vi "Copilot-Screen-(Controller).vi"() -> ()   [LabVIEW 2018]
uses:
  <vilib>/Instr/_visa.llb/VISA Configure Serial Port (Instr).vi
  <vilib>/Utility/inputDevices.llb/joystickAcquire.vi
  <vilib>/Utility/inputDevices.llb/closeJoystick.vi
  <vilib>/MakerHub/LINX/LMH-LINX.lvlib
panel:
  out "PH Reading":dbl format="%#_2f"
  in  "Horizontal Pulse 2":i32 caption="mp"
  out "Loop Rate (Hz)":u32
  in  "Temperature":bool
  in  "PH":bool
  in  "Metal":bool
  in  "R7":bool
  in  "R8":bool
  out "U Scaled":i32
  out "Teather Motor":bool
  out "Micro Backward":bool
  out "Micro Right":bool
  out "Micro Left":bool
  out "Micro Forward":bool
  out "CW":bool
  out "CCW":bool
  in  "MLED":bool
  in  "LMB":bool
  in  "LMF":bool
  in  "RMB":bool
  in  "RMF":bool
  in  "Reset":bool
  out "Seconds":i32
  out "Minutes":i32
  out "Timeout?":bool
  out "Horse Forward":bool
  out "Horse Backward":bool
  out "Down":bool
  out "Up":bool
  out "Backward":bool
  out "Left":bool
  out "Right":bool
  out "Forward":bool
  out "Horizontal Motion Case":string
  out "Horizontal %":i32
  out "Vertical Motion Case":string
  out "Vertical %":i32
  in  "Emergency Stop":bool
  out "X Scaled":i32
  out "Y Scaled":i32
  out "Z Scaled":i32
  out "ZR Scaled":i32
  out "axis info":T1
  out "button info":T2
  out "direction info":T3
  in  "R1":bool
  in  "ARM":bool
  in  "R3":bool
  in  "R4":bool
  in  "T1":bool
  in  "T2":bool
  in  "motion front left":bool
  in  "motion front right":bool
  in  "motion back right":bool
  in  "motion back left":bool
  in  "vertica front motors dir":bool
  in  "vertical back motors dir":bool
  in  "Horizontal Pulse 1":i32 caption="mp"
  in  "Vertical Pulse":i32 caption="vp"
  in  "To Arduino":string caption="Result"
  out "Sensor Reading":string
  out "error out":errorcluster
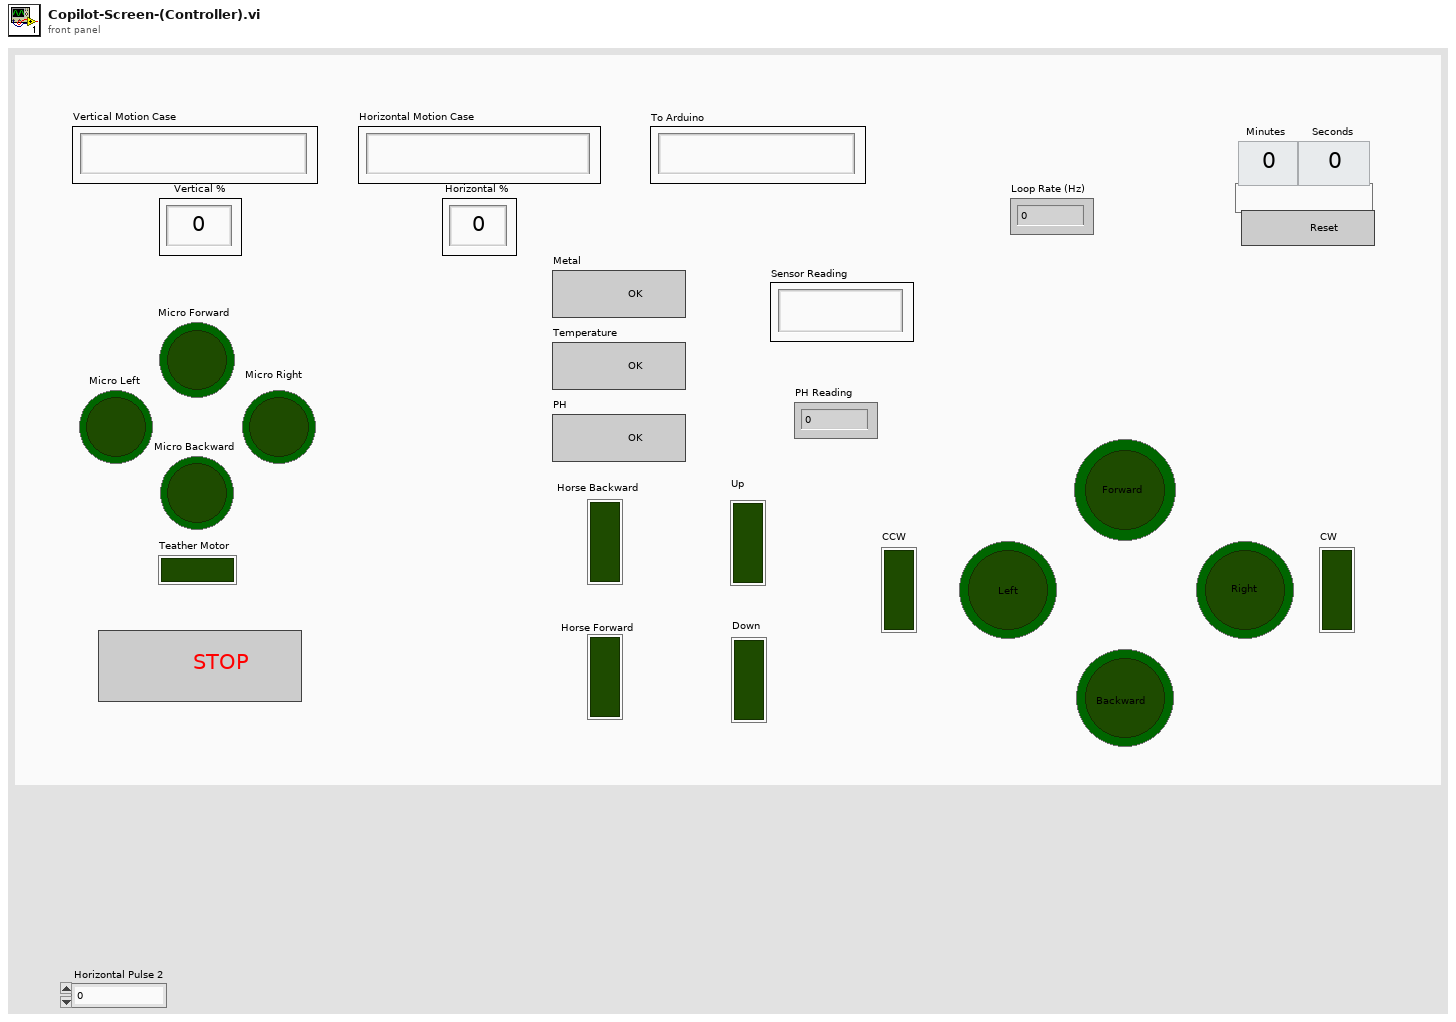
[diagram p1: front panel]
types:
  T1 = cluster{"X axis":i32, "Y axis":i32, "Z axis":i32, "X axis rotation":i32, "Y axis rotation":i32, "Z axis rotation":i32, "U axis":i32, "V axis":i32}
  T2 = cluster{"button 1":bool, "button 2":bool, "button 3":bool, "button 4":bool, "button 5":bool, "button 6":bool, "button 7":bool, "button 8":bool, "button 9":bool, "button 10":bool, "button 11":bool, "button 12":bool, "button 13":bool, "button 14":bool, "button 15":bool, "button 16":bool, "button 17":bool, "button 18":bool, "button 19":bool, "button 20":bool, "button 21":bool, "button 22":bool, "button 23":bool, "button 24":bool, "button 25":bool, "button 26":bool, "button 27":bool, "button 28":bool, "button 29":bool, "button 30":bool, "button 31":bool, "button 32":bool}
  T3 = cluster{"pov 1":i32, "pov 2":i32, "pov 3":i32, "pov 4":i32}
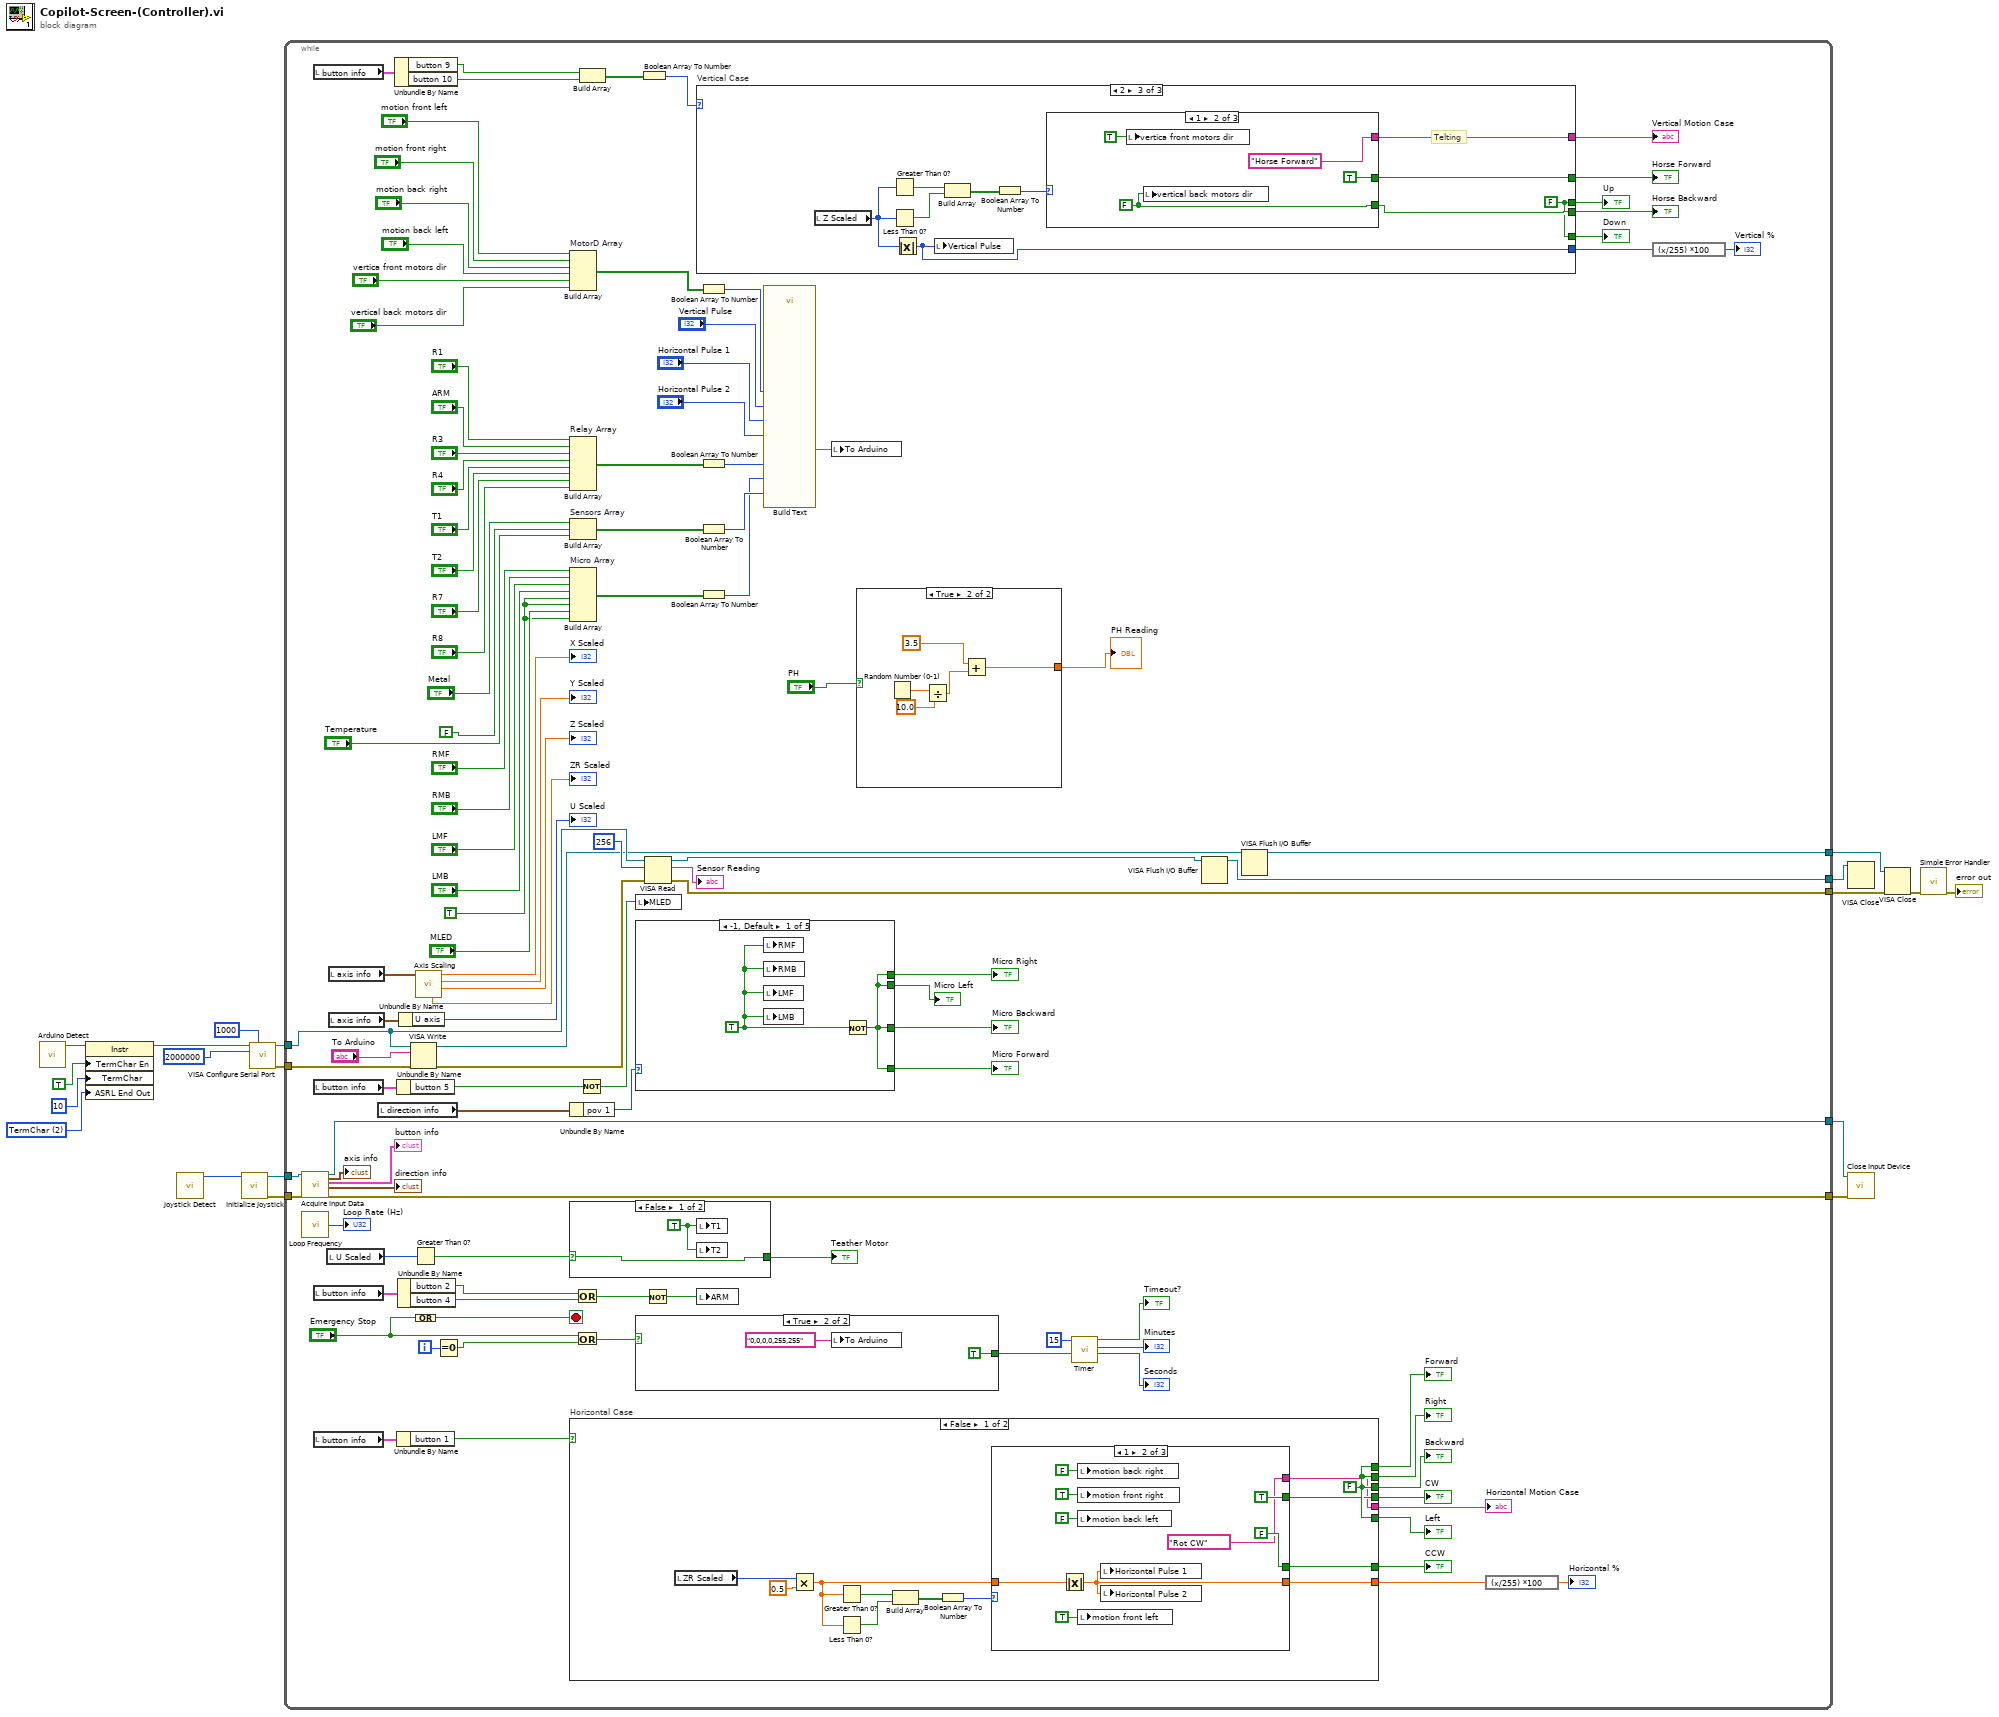
[diagram p0: block diagram]
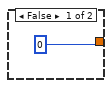
[diagram p2: hidden frame]
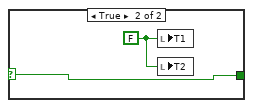
[diagram p3: hidden frame]
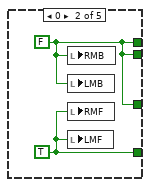
[diagram p4: hidden frame]
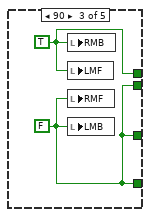
[diagram p5: hidden frame]
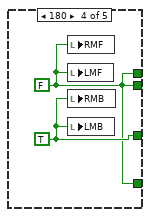
[diagram p6: hidden frame]
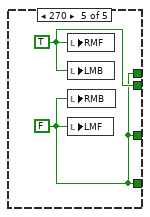
[diagram p7: hidden frame]
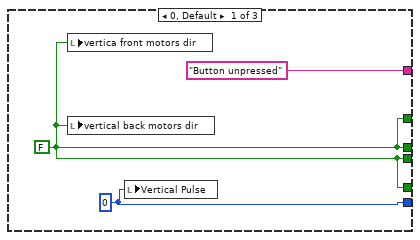
[diagram p8: hidden frame]
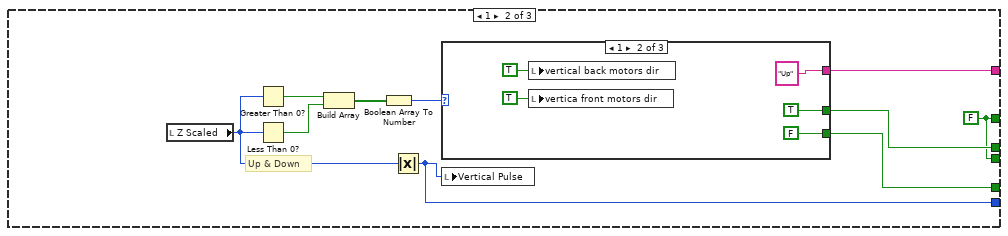
[diagram p9: hidden frame]
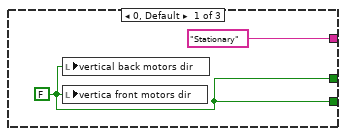
[diagram p10: hidden frame]
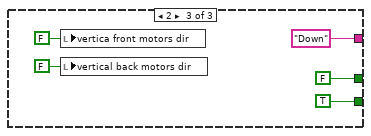
[diagram p11: hidden frame]
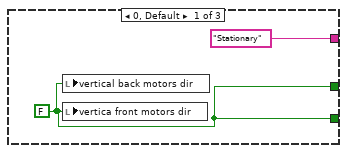
[diagram p12: hidden frame]
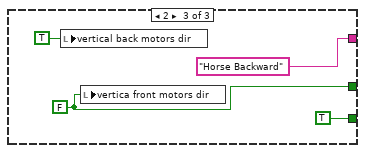
[diagram p13: hidden frame]
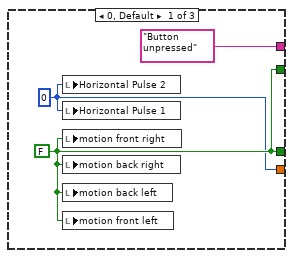
[diagram p14: hidden frame]
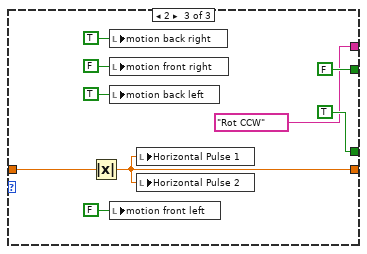
[diagram p15: hidden frame]
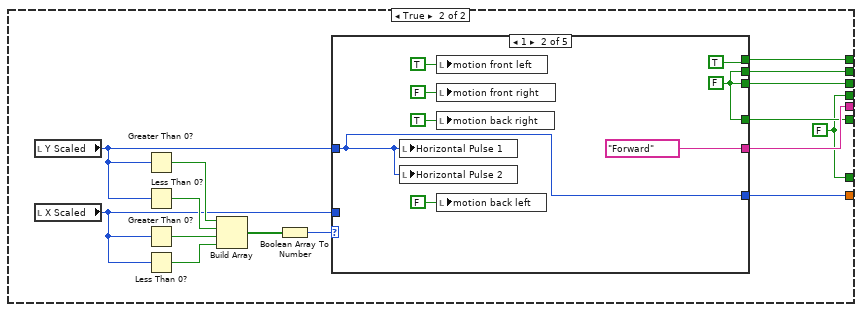
[diagram p16: hidden frame]
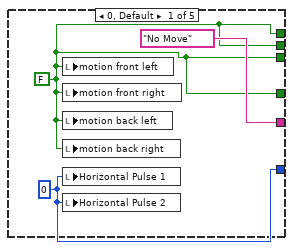
[diagram p17: hidden frame]
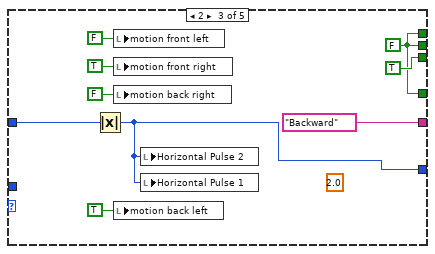
[diagram p18: hidden frame]
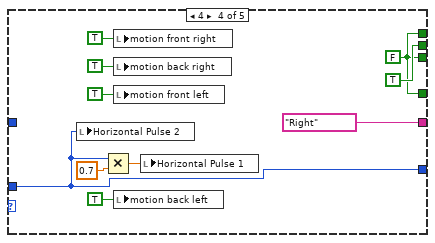
[diagram p19: hidden frame]
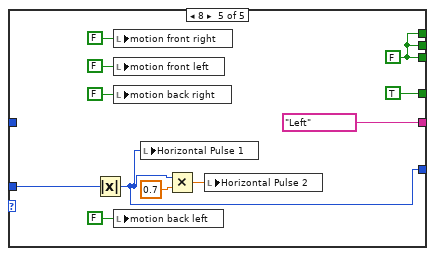
[diagram p20: hidden frame]
diagram:
  w5 = u16 2 items=["None", "Last Bit", "TermChar", "Break"] ("Serial Settings:End Mode for Writes")
  n1 = call "Arduino Detect.vi"() -> ("VISA Refnum out"=w2:refnum<visa-resource-name>)  [unwired: 9 in, 2 out]
  n2 = property class="Instr"(reference=w2, "TermChar En"=TRUE ("Message Based Settings:Termination Character Enable"), "TermChar"=u8 10 ("Message Based Settings:Termination Character"), "ASRL End Out"=w5) -> (reference out=w3:refnum<visa-resource-name>)  [unwired: 1 in, 1 out]
  n3 = call "Joystick Detect.vi"() -> ("ID"=w1:i32)  [unwired: 11 in]
  n4 = call <vilib>:"Initialize Joystick.vi"("device index"=w1) -> ("error out"=w10:errorcluster, "device ID"=w11:refnum<k1>)  [unwired: 9 in]
  n5 = call-poly "VISA Configure Serial Port"("VISA resource name"=w3, "timeout (10sec)"=u32 1000, "baud rate (9600)"=u32 2000000 ("baud rate")) -> ("VISA resource name out"=w15:refnum<visa-resource-name>, "error out"=w14:errorcluster)  [unwired: 11 in]
  n6 = while {
    tunnel: w15 -> [w88]
    tunnel: w14 -> [w130]
    tunnel: [w87] -> w13
    tunnel: [w129] -> w12
    tunnel: w11 -> [w111]
    tunnel: w10 -> [w110]
    tunnel: [w109] -> w9
    tunnel: [w108] -> w8
    tunnel: [w79] -> w7
    i -> [w85]
    stop <- w104 stop-if-true
    w23 = TRUE
    n7 = call-poly <vilib>:"Acquire Input Data.vi"("device ID"=w111, "error in (no error)"=w110) -> ("device ID"=w108:refnum<k1>, "axis info"=→"axis info":T1, "button info"=→"button info":T2, "direction info"=→"direction info":T3, "error out"=w109:errorcluster)  [unwired: 13 in]
    n8 = call <vilib>:"Loop Frequency.vi"() -> ("Loop Rate (Hz)"=→"Loop Rate (Hz)":u32)
    n9 = local read "button info"() -> (w100:T2)
    n10 = local read "button info"() -> (w44:T2)
    n11 = local read "button info"() -> (w89:T2)
    n12 = local read "button info"() -> (w93:T2)
    n13 = local read "U Scaled"() -> (w49:i32)
    n14 = local read "axis info"() -> (w74:T1)
    n15 = local read "axis info"() -> (w40:T1)
    n16 = local read "direction info"() -> (w59:T3)
    n17 = Unbundle By Name(w100) -> ("button 9"=w99:bool, "button 10"=w98:bool)
    n18 = Unbundle By Name(w44) -> ("button 5"=w43:bool)
    n19 = Unbundle By Name(w93) -> ("button 1"=w53:bool)
    n20 = Unbundle By Name(w89) -> ("button 2"=w82:bool, "button 4"=w81:bool)
    n21 = Unbundle By Name(w40) -> ("U axis"=→"U Scaled":i32)
    n22 = VISA Write(VISA resource name=w88, write buffer="To Arduino", error in (no error)=w130) -> (VISA resource name out=w86:refnum<visa-resource-name>, error out=w132:errorcluster)  [unwired: 1 out]
    n23 = Greater Than 0?(x=w49) -> (x > 0?=w46:bool)
    n24 = call "Axis Scaling.vi"("axis info"=w74) -> ("Scalar 2"=→"Z Scaled":dbl, "Scalar"=→"Y Scaled":dbl, "Scalar 4"=→"X Scaled":dbl, "Scalar 3"=→"ZR Scaled":dbl)  [unwired: 6 in, 1 out]
    n25 = Compound Arithmetic op=OR("Emergency Stop") -> (w104:bool)
    n26 = Equal To 0?(x=w85) -> (x = 0?=w105:bool)
    n27 = Build Array "MotorD Array"("motion front left", "motion front right", "motion back right", "motion back left", "vertica front motors dir", "vertical back motors dir") -> (w126:bool[])
    n28 = Build Array "Relay Array"("R1", "ARM", "R3", "R4", "T1", "T2", "R7", "R8") -> (w118:bool[])
    n29 = Build Array "Sensors Array"("Metal", FALSE ("element"), "Temperature") -> (w38:bool[])
    n30 = Build Array "Micro Array"("RMF", "RMB", "LMF", "LMB", w23, w23, "MLED", w23) -> (w29:bool[])
    n31 = Unbundle By Name(w59) -> ("pov 1"=w58:i32)
    n32 = case shown="False" w46 {
      selector: w46 -> [w140 w142]
      tunnel: [w140 w142] -> w45
      frame False {
        w139 = TRUE ("LMF")
        n33 = local write "T1"(w139) -> ()
        n34 = local write "T2"(w139) -> ()
      }
      frame True {
        w141 = FALSE ("LMF")
        n35 = local write "T1"(w141) -> ()
        n36 = local write "T2"(w141) -> ()
      }
    }
    "Teather Motor" <- w45
    n37 = case "Horizontal Case" shown="False" w53 {
      tunnel: [w201 w245] -> w96
      tunnel: [w202 w236] -> w95
      tunnel: [w209 w234] -> w64
      tunnel: [w209 w233] -> w63
      tunnel: [w209 w232] -> w62
      tunnel: [w209 w235] -> w61
      tunnel: [w204 w231] -> w52
      tunnel: [w203 w231] -> w51
      frame False {
        w209 = FALSE ("motion back left")
        n38 = local read "ZR Scaled"() -> (w200:i32)
        n39 = Multiply(x=w200, y=0.5) -> (x*y=w199:dbl)
        n40 = Greater Than 0?(x=w199) -> (x > 0?=w207:bool)
        n41 = Less Than 0?(x=w199) -> (x < 0?=w208:bool)
        n42 = Build Array(w207, w208) -> (w205:bool[])
        n43 = Boolean Array To Number(Boolean array=w205) -> (number=w206:u32)
        n44 = case shown="1" w206 {
          tunnel: [w210 w213 w222] -> w202
          tunnel: [w212 FALSE TRUE] -> w204
          tunnel: [w212 TRUE FALSE] -> w203
          tunnel: w199 -> [_ w215 w224]
          tunnel: ["Button unpressed" ("String 2") "Rot CW" ("String 2") "Rot CCW" ("String 2")] -> w201
          frame 0, Default {
            w212 = FALSE
            w210 = 0 ("Motion Pulse")
            n45 = local write "Horizontal Pulse 2"(w210) -> ()
            n46 = local write "Horizontal Pulse 1"(w210) -> ()
            n47 = local write "motion front right"(w212) -> ()
            n48 = local write "motion back right"(w212) -> ()
            n49 = local write "motion back left"(w212) -> ()
            n50 = local write "motion front left"(w212) -> ()
          }
          frame 1 {
            n51 = Absolute Value(x=w215) -> (abs(x)=w213:dbl)
            n52 = local write "motion back right"(FALSE) -> ()
            n53 = local write "motion front right"(TRUE) -> ()
            n54 = local write "motion back left"(FALSE) -> ()
            n55 = local write "motion front left"(TRUE) -> ()
            n56 = local write "Horizontal Pulse 1"(w213) -> ()
            n57 = local write "Horizontal Pulse 2"(w213) -> ()
          }
          frame 2 {
            n58 = Absolute Value(x=w224) -> (abs(x)=w222:dbl)
            n59 = local write "motion back right"(TRUE) -> ()
            n60 = local write "motion front right"(FALSE) -> ()
            n61 = local write "motion back left"(TRUE) -> ()
            n62 = local write "motion front left"(FALSE) -> ()
            n63 = local write "Horizontal Pulse 1"(w222) -> ()
            n64 = local write "Horizontal Pulse 2"(w222) -> ()
          }
        }
      }
      frame True {
        w231 = FALSE ("motion back left")
        n65 = local read "Y Scaled"() -> (w238:i32)
        n66 = local read "X Scaled"() -> (w237:i32)
        n67 = Greater Than 0?(x=w238) -> (x > 0?=w243:bool)
        n68 = Less Than 0?(x=w238) -> (x < 0?=w242:bool)
        n69 = Greater Than 0?(x=w237) -> (x > 0?=w241:bool)
        n70 = Less Than 0?(x=w237) -> (x < 0?=w240:bool)
        n71 = Build Array(w243, w242, w241, w240) -> (w239:bool[])
        n72 = Boolean Array To Number(Boolean array=w239) -> (number=w244:u32)
        n73 = case shown="1" w244 {
          tunnel: ["No Move" ("String 2") "Forward" ("String 2") "Backward" ("String 2") "Right" ("String 2") "Left" ("String 2")] -> w245
          tunnel: w238 -> [_ w249 w264 _ _]
          tunnel: w237 -> [_ _ _ w267 w285]
          tunnel: [w246 w249 w257 w267 w276] -> w236
          tunnel: [w247 w250 w258 w269 TRUE] -> w235
          tunnel: [w247 w250 TRUE w269 w279] -> w234
          tunnel: [w247 TRUE w258 w269 w279] -> w233
          tunnel: [w247 w250 w258 TRUE w279] -> w232
          frame 0, Default {
            w247 = FALSE
            w246 = 0 ("Motion Pulse")
            n74 = local write "motion front left"(w247) -> ()
            n75 = local write "motion front right"(w247) -> ()
            n76 = local write "motion back left"(w247) -> ()
            n77 = local write "motion back right"(w247) -> ()
            n78 = local write "Horizontal Pulse 1"(w246) -> ()
            n79 = local write "Horizontal Pulse 2"(w246) -> ()
          }
          frame 1 {
            w250 = FALSE
            n80 = local write "Horizontal Pulse 1"(w249) -> ()
            n81 = local write "Horizontal Pulse 2"(w249) -> ()
            n82 = local write "motion front left"(TRUE) -> ()
            n83 = local write "motion front right"(FALSE) -> ()
            n84 = local write "motion back right"(TRUE) -> ()
            n85 = local write "motion back left"(FALSE) -> ()
          }
          frame 2 {
            (unwired) 2.0 ("y")
            w258 = FALSE
            n86 = Absolute Value(x=w264) -> (abs(x)=w257:i32)
            n87 = local write "motion front left"(FALSE) -> ()
            n88 = local write "motion front right"(TRUE) -> ()
            n89 = local write "motion back right"(FALSE) -> ()
            n90 = local write "motion back left"(TRUE) -> ()
            n91 = local write "Horizontal Pulse 2"(w257) -> ()
            n92 = local write "Horizontal Pulse 1"(w257) -> ()
          }
          frame 4 {
            w269 = FALSE
            n93 = local write "Horizontal Pulse 2"(w267) -> ()
            n94 = Multiply(x=w267, y=0.7) -> (x*y=w266:dbl)
            n95 = local write "motion front right"(TRUE) -> ()
            n96 = local write "motion back right"(TRUE) -> ()
            n97 = local write "motion front left"(TRUE) -> ()
            n98 = local write "motion back left"(TRUE) -> ()
            n99 = local write "Horizontal Pulse 1"(w266) -> ()
          }
          frame 8 {
            w279 = FALSE
            n100 = Absolute Value(x=w285) -> (abs(x)=w276:i32)
            n101 = local write "motion front right"(FALSE) -> ()
            n102 = local write "motion front left"(FALSE) -> ()
            n103 = local write "motion back right"(FALSE) -> ()
            n104 = local write "motion back left"(FALSE) -> ()
            n105 = local write "Horizontal Pulse 1"(w276) -> ()
            n106 = Multiply(x=w276, y=0.7) -> (x*y=w277:dbl)
            n107 = local write "Horizontal Pulse 2"(w277) -> ()
          }
        }
      }
    }
    "Horizontal Motion Case" <- w96
    "Forward" <- w63
    "Right" <- w62
    "Left" <- w61
    "Backward" <- w64
    "CCW" <- w52
    "CW" <- w51
    n108 = Or(x=w82, y=w81) -> (x .or. y?=w60:bool)
    n109 = Or(x="Emergency Stop", y=w105) -> (x .or. y?=w107:bool)
    n110 = Not(x=w43) -> (.not. x?=w42:bool)
    n111 = Build Array(w99, w98) -> (w97:bool[])
    n112 = local write "MLED"(w42) -> ()
    n113 = case shown="-1, Default" w58 {
      tunnel: [w143 w146 w147 w149 w151] -> w57
      tunnel: [w143 w145 w148 w149 w151] -> w56
      tunnel: [w143 w145 w147 w150 w151] -> w55
      tunnel: [w143 w145 w147 w149 w152] -> w54
      frame -1, Default {
        w144 = TRUE ("RMF")
        n114 = local write "RMF"(w144) -> ()
        n115 = local write "RMB"(w144) -> ()
        n116 = local write "LMF"(w144) -> ()
        n117 = local write "LMB"(w144) -> ()
        n118 = Not(x=w144) -> (.not. x?=w143:bool)
      }
      frame 0 {
        w145 = FALSE ("RMF")
        w146 = TRUE ("RMF")
        n119 = local write "RMB"(w145) -> ()
        n120 = local write "LMB"(w145) -> ()
        n121 = local write "RMF"(w146) -> ()
        n122 = local write "LMF"(w146) -> ()
      }
      frame 90 {
        w147 = FALSE ("RMF")
        w148 = TRUE ("LMF")
        n123 = local write "RMB"(w148) -> ()
        n124 = local write "LMF"(w148) -> ()
        n125 = local write "RMF"(w147) -> ()
        n126 = local write "LMB"(w147) -> ()
      }
      frame 180 {
        w149 = FALSE ("LMF")
        w150 = TRUE ("RMB")
        n127 = local write "RMF"(w149) -> ()
        n128 = local write "LMF"(w149) -> ()
        n129 = local write "RMB"(w150) -> ()
        n130 = local write "LMB"(w150) -> ()
      }
      frame 270 {
        w151 = FALSE ("RMB")
        w152 = TRUE ("RMF")
        n131 = local write "RMF"(w152) -> ()
        n132 = local write "LMB"(w152) -> ()
        n133 = local write "RMB"(w151) -> ()
        n134 = local write "LMF"(w151) -> ()
      }
    }
    "Micro Forward" <- w57
    "Micro Left" <- w54
    "Micro Right" <- w56
    "Micro Backward" <- w55
    n135 = case shown="True" w107 {
      tunnel: ["Reset" TRUE ("Reset")] -> w69
      frame False {
      }
      frame True {
        n136 = local write "To Arduino"("0,0,0,0,255,255" ("write string")) -> ()
      }
    }
    n137 = Boolean Array To Number(Boolean array=w97) -> (number=w83:u32)
    n138 = VISA Read(VISA resource name=w88, byte count=u32 256, error in (no error)=w132) -> (VISA resource name out=w80:refnum<visa-resource-name>, read buffer=→"Sensor Reading":string, error out=w129:errorcluster)  [unwired: 1 out]
    n139 = Not(x=w60) -> (.not. x?=w50:bool)
    n140 = case "Vertical Case" shown="2" w83 {
      tunnel: ["Button unpressed" ("String 3") w164 w182] -> w103
      tunnel: [w154 w163 w181] -> w102
      tunnel: [w153 w158 w178] -> w78
      tunnel: [w153 w157 w178] -> w77
      tunnel: [w153 w156 w180] -> w76
      tunnel: [w153 w156 w179] -> w75
      frame 0, Default {
        w153 = FALSE ("vertica front motors dir")
        w154 = 0 ("Vertical Pulse")
        n141 = local write "vertica front motors dir"(w153) -> ()
        n142 = local write "vertical back motors dir"(w153) -> ()
        n143 = local write "Vertical Pulse"(w154) -> ()
      }
      frame 1 {
        w156 = FALSE ("Up")
        # "Up & Down"
        n144 = local read "Z Scaled"() -> (w159:i32)
        n145 = Greater Than 0?(x=w159) -> (x > 0?=w160:bool)
        n146 = Less Than 0?(x=w159) -> (x < 0?=w161:bool)
        n147 = Build Array(w160, w161) -> (w162:bool[])
        n148 = Boolean Array To Number(Boolean array=w162) -> (number=w165:u32)
        n149 = Absolute Value(x=w159) -> (abs(x)=w163:i32)
        n150 = case shown="1" w165 {
          tunnel: ["Stationary" ("f") "Up" ("String 3") "Down" ("String 3")] -> w164
          tunnel: [w166 TRUE ("Up") FALSE ("Down")] -> w158
          tunnel: [w166 FALSE ("Up") TRUE ("Down")] -> w157
          frame 0, Default {
            w166 = FALSE ("vertica front motors dir")
            n151 = local write "vertical back motors dir"(w166) -> ()
            n152 = local write "vertica front motors dir"(w166) -> ()
          }
          frame 1 {
            n153 = local write "vertical back motors dir"(TRUE ("vertica front motors dir")) -> ()
            n154 = local write "vertica front motors dir"(TRUE ("vertica front motors dir")) -> ()
          }
          frame 2 {
            n155 = local write "vertica front motors dir"(FALSE ("vertica front motors dir")) -> ()
            n156 = local write "vertical back motors dir"(FALSE ("vertical back motors dir")) -> ()
          }
        }
        n157 = local write "Vertical Pulse"(w163) -> ()
      }
      frame 2 {
        w178 = FALSE ("vertica front motors dir")
        # "Telting"
        n158 = local read "Z Scaled"() -> (w187:i32)
        n159 = Greater Than 0?(x=w187) -> (x > 0?=w185:bool)
        n160 = Less Than 0?(x=w187) -> (x < 0?=w184:bool)
        n161 = Absolute Value(x=w187) -> (abs(x)=w181:i32)
        n162 = local write "Vertical Pulse"(w181) -> ()
        n163 = Build Array(w185, w184) -> (w183:bool[])
        n164 = Boolean Array To Number(Boolean array=w183) -> (number=w186:u32)
        n165 = case shown="1" w186 {
          tunnel: ["Stationary" ("f") "Horse Forward" ("String 3") "Horse Backward" ("String 3")] -> w182
          tunnel: [w188 TRUE ("Horse Forward") w194] -> w180
          tunnel: [w188 w190 TRUE ("Horse Backward")] -> w179
          frame 0, Default {
            w188 = FALSE ("vertica front motors dir")
            n166 = local write "vertical back motors dir"(w188) -> ()
            n167 = local write "vertica front motors dir"(w188) -> ()
          }
          frame 1 {
            w190 = FALSE ("vertica front motors dir")
            n168 = local write "vertica front motors dir"(TRUE ("vertica front motors dir")) -> ()
            n169 = local write "vertical back motors dir"(w190) -> ()
          }
          frame 2 {
            w194 = FALSE ("vertica front motors dir")
            n170 = local write "vertical back motors dir"(TRUE ("vertica front motors dir")) -> ()
            n171 = local write "vertica front motors dir"(w194) -> ()
          }
        }
      }
    }
    "Vertical Motion Case" <- w103
    "Up" <- w78
    "Down" <- w77
    "Horse Forward" <- w76
    "Horse Backward" <- w75
    n172 = local write "ARM"(w50) -> ()
    n173 = Boolean Array To Number(Boolean array=w126) -> (number=w31:u32)
    n174 = Boolean Array To Number(Boolean array=w118) -> (number=w32:u32)
    n175 = Boolean Array To Number(Boolean array=w38) -> (number=w34:u32)
    n176 = Boolean Array To Number(Boolean array=w29) -> (number=w33:u32)
    n177 = call "Build Text"("MotorD"=w31, "Micro"=w33, "VP"="Vertical Pulse", "HP1"="Horizontal Pulse 1", "HP2"="Horizontal Pulse 2", "Relay"=w32, "Sensors"=w34) -> ("Result"=w92:string)  [unwired: 7 in, 1 out]
    n178 = local write "To Arduino"(w92) -> ()
    n179 = case shown="True" "PH" {
      tunnel: [0 w134] -> w20
      frame False {
      }
      frame True {
        n180 = Random Number (0-1)() -> (number: 0 to 1=w136:dbl)
        n181 = Divide(x=w136, y=10.0) -> (x/y=w137:dbl)
        n182 = Add(x=3.5, y=w137) -> (x+y=w134:dbl)
      }
    }
    "PH Reading" <- w20
    n183 = call "Timer.vi"("My Minutes"=15, "Reset"=w69) -> ("Timeout?"=→"Timeout?":bool, "Minutes"=→"Minutes":i32, "Seconds"=→"Seconds":i32)  [unwired: 6 in]
    n184 = VISA Flush I/O Buffer(VISA resource name=w80) -> (VISA resource name out=w79:refnum<visa-resource-name>)  [unwired: 2 in, 1 out]
    n185 = VISA Flush I/O Buffer(VISA resource name=w86) -> (VISA resource name out=w87:refnum<visa-resource-name>)  [unwired: 2 in, 1 out]
    n186 = expression code="(x/255) *100"(w95) -> (→"Horizontal %":dbl)
    n187 = expression code="(x/255) *100"(w102) -> (→"Vertical %":i32)
  }
  n188 = VISA Close(VISA resource name=w7) -> ()  [unwired: 1 in, 1 out]
  n189 = call-poly <vilib>:"Close Input Device.vi"("error in (no error)"=w9, "device ID"=w8) -> ()  [unwired: 8 in, 1 out]
  n190 = VISA Close(VISA resource name=w13, error in (no error)=w12) -> (error out=w18:errorcluster)
  n191 = call <vilib>:"Simple Error Handler.vi"("error in (no error)"=w18) -> ("error out"=→"error out":errorcluster)  [unwired: 4 in, 4 out]
